vi "Server_Emails.vi"(0 "Client Name Contains":string, 1 "Message":string, 2 "Contact All clients?":bool, 3 "Subject":string, 4 "Extra People to Email":string[](array[string])) -> ()   [LabVIEW 2010]
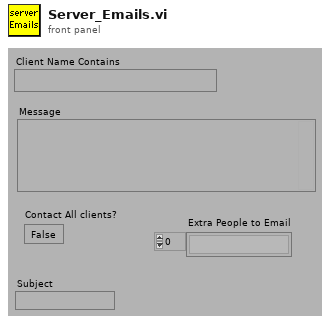
[diagram p1: front panel]
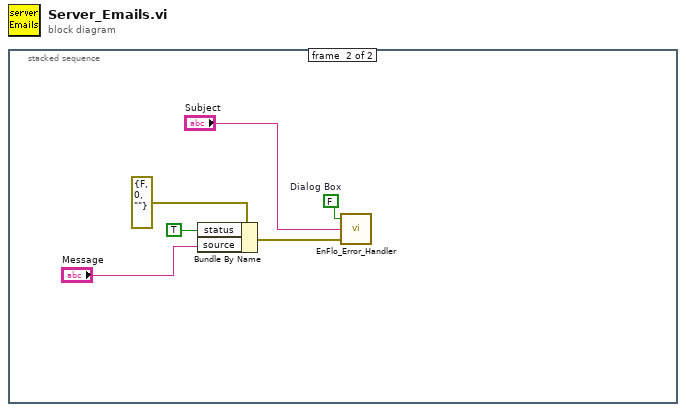
[diagram p0: block diagram]
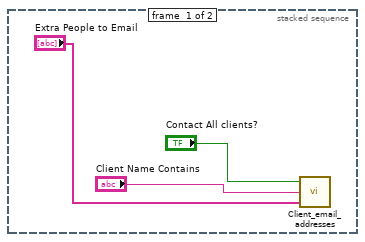
[diagram p2: hidden frame]
diagram:
  n1 = stacked-sequence {
    frame #0 {
      n2 = call "Client_email_addresses.vi"("Extra People to Email"="Extra People to Email", "Client Name Contains"="Client Name Contains", "Contact All clients?"="Contact All clients?") -> ()
    }
    frame #1 {
      w5 = FALSE  # Dialog Box
      n3 = Bundle By Name(cluster=errorcluster {"status"=FALSE, "code"=0, "source"=""} ("error in (no error)"), "status"=TRUE ("Bundle Element"), "source"="Message") -> (w7:errorcluster)
      n4 = call "EnFlo_Error_Handler.vi"("error in (no error)"=w7, "Error Type"="Subject", "Dialog Box (T)"=w5) -> ()  [unwired: 3 out]
    }
  }
